vi "Load Resource File.vi"(8 "error in (no error)":errorcluster, 11 "Resource file":path) -> (0 "error out":errorcluster, 2 "File Type":string, 3 "Resources":T1)   [LabVIEW 2017]
uses:
  Resource Array.ctl
  Resource.ctl
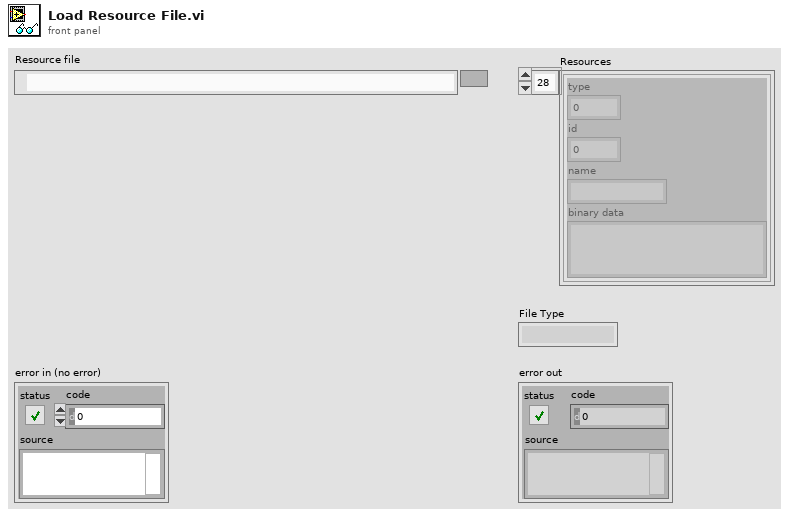
[diagram p1: front panel]
types:
  T1 = typedef "Resource Array.ctl" = T2[]
  T2 = typedef "Resource.ctl" = cluster{"type":u32, "id":i32, "name":string, "binary data":string}
  T3 = cluster{"type":u32, "id":i32, "name":string, "binary data":string}[]
  T4 = cluster{"type":u32, "id":i32, "name":string, "binary data":string}
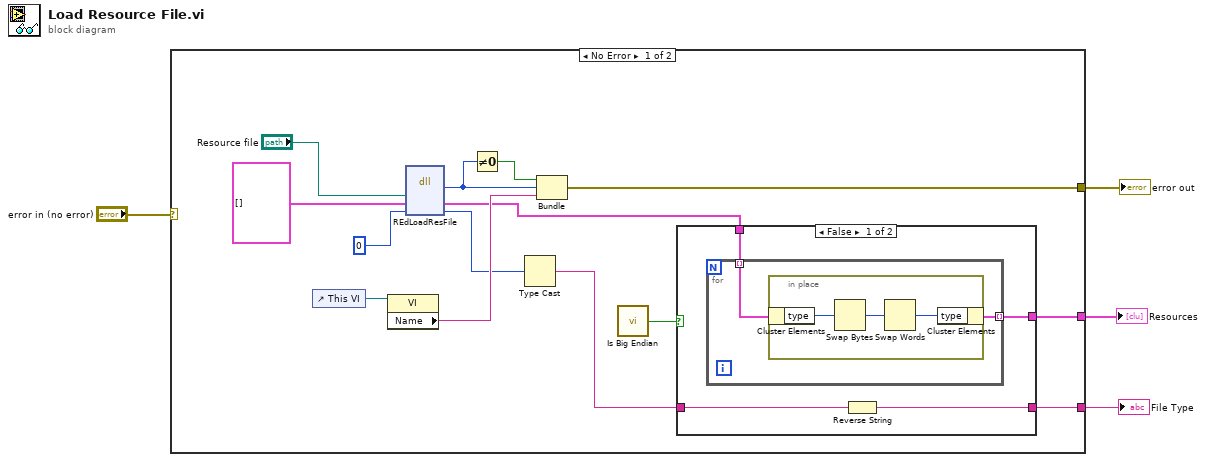
[diagram p0: block diagram]
diagram:
  n1 = case shown="No Error" "error in (no error)" {
    selector: "error in (no error)" -> [_ w30]
    tunnel: [w10 w30] -> w4
    tunnel: [w8 _] -> w2
    tunnel: [w7 _] -> w1
    frame No Error {
      n2 = control-ref of="This VI"() -> (w15:refnum<vi>)
      n3 = property class="VI"(reference=w15) -> ("Name"=w12:string)  [unwired: 1 in, 2 out]
      n4 = dll-call lib="LabVIEW" fn="REdLoadResFile"("resource binary file"="Resource file", "resources"=T3 [], 0) -> (w14:i32, "resources"=w9:T3, w11:i32)  [unwired: 4 in, 2 out]
      n5 = Not Equal To 0?(x=w14) -> (x != 0?=w13:bool)
      n6 = Type Cast(x=w11) -> (*(type *) &x=w6:string)  [unwired: 1 in]
      n7 = Bundle(w13, w14, "Name"=w12) -> (w10:cluster{bool, i32, "Name":string})  [unwired: 1 in]
      n8 = call "Is Big Endian.vi"() -> ("big endian"=w5:bool)
      n9 = case shown="False" w5 {
        tunnel: w9 -> [w22 w29]
        tunnel: [w21 w29] -> w8
        tunnel: [w19 w28] -> w7
        tunnel: w6 -> [w20 w28]
        frame False {
          n10 = for {
            tunnel: w22 -> [w24] mode=indexing
            tunnel: [w23] -> w21 mode=indexing
            n11 = in-place {
              n12 = in-place-cluster #1(w24) -> ("type"=w27:u32)
              n13 = Swap Bytes(anything=w27) -> (byte swapped=w26:u32)
              n14 = Swap Words(1:w26) -> (0:w25:u32)
              n15 = in-place-cluster #1("type"=w25) -> (w23:T4)
            }
          }
          n16 = Reverse String(1:w20) -> (0:w19:string)
        }
        frame True {
        }
      }
    }
    frame Error {
    }
  }
  "error out" <- w4
  "Resources" <- w2
  "File Type" <- w1
